vi "Skew.vi"(1 "k":dbl[](array[numeric])) -> (0 "M":T1)   [LabVIEW 2013, in "Finger.lvclass"]
uses:
  Finger.lvclass
  <vilib>/Analysis/Matrix/Datatypes/RealMatrix.ctl
  <vilib>/Analysis/Matrix/NI_Matrix.lvlib
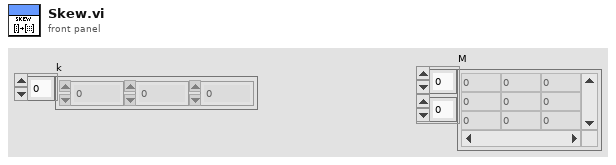
[diagram p1: front panel]
types:
  T1 = typedef "NI_Matrix.lvlib/RealMatrix.ctl" = dbl[][]
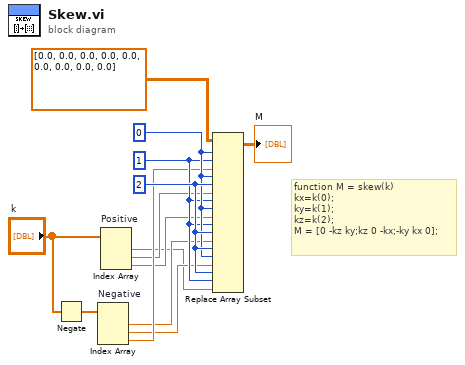
[diagram p0: block diagram]
diagram:
  w9 = 2 ("disabled index (row)")
  w7 = 1 ("disabled index (row)")
  w8 = 0 ("disabled index (row)")
  # "function M = skew(k)\nkx=k(0);\nky=k(1);\nkz=k(2);\nM = [0 -kz ky;kz 0 -kx;-ky kx 0];"
  n1 = Negate(x="k") -> (-x=w12:dbl[])
  n2 = Index Array "Negative"(array=w12) -> (element #1=w3:dbl, element #2=w2:dbl, element #3=w6:dbl)  [unwired: 3 in]
  n3 = Index Array "Positive"(array="k") -> (element #1=w1:dbl, element #2=w5:dbl, element #3=w4:dbl)  [unwired: 3 in]
  n4 = Replace Array Subset(array=T1 [[0.0, 0.0, 0.0], [0.0, 0.0, 0.0], [0.0, 0.0, 0.0]] ("matrix"), new element #1=w6, index (row) #1=w8, index (col) #1=w7, new element #2=w5, index (row) #2=w8, index (col) #2=w9, new element #3=w4, index (row) #3=w7, index (col) #3=w8, new element #4=w3, index (row) #4=w7, index (col) #4=w9, new element #5=w2, index (row) #5=w9, index (col) #5=w8, new element #6=w1, index (row) #6=w9, index (col) #6=w7) -> (→"M":T1)
